vi "get system trace.vi"(6 "Amplifier":T1(ring), 7 "Attenuator":enum16{"NA", "6dB-ME811 "}(ring), 8 "Cable 3":enum16{"NA", "ME1249", "ME1245", "ME1244"}(ring), 9 "Cable 2":enum16{"NA", "ME1249", "ME1245", "ME1244"}(ring), 10 "Cable 1":enum16{"NA", "ME1249", "ME1245", "ME1244"}(ring), 11 "Antenna":T2(ring)) -> (0 "Nuber of Points":i32, 2 "Corrected System Trace":cluster{dbl[], "x+y":dbl[]}, 3 "Corrected 2D array":dbl[][](array[numeric]))   [LabVIEW 2016]
doc: "This VI generate corrected plot of measurement system adding up antenna factor, cable loss, attenuation and amplification along the way."
panel:
  out "Stop Frequency":dbl
  out "Start Frequency":dbl
  out "XY Graph":cluster{dbl[], "x+y":dbl[]}(graph)
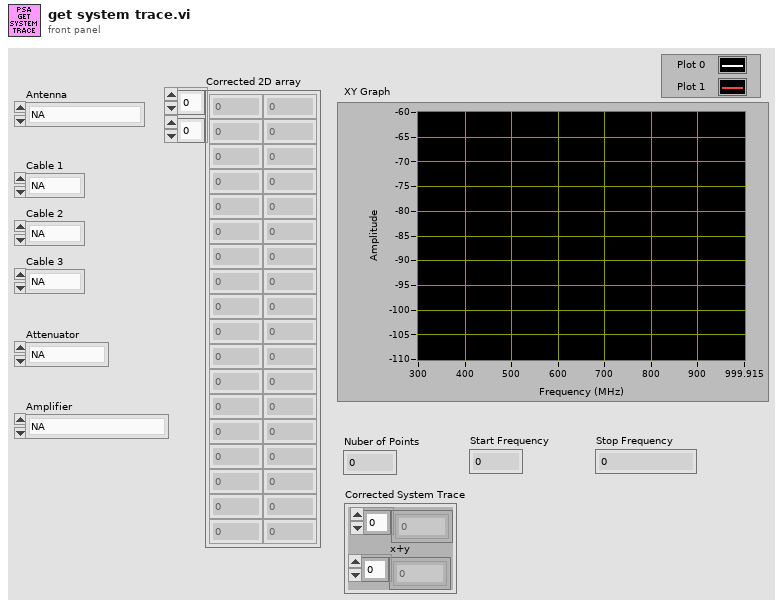
[diagram p1: front panel]
types:
  T1 = enum16{"NA", "500M-18GHz-ME1241", "10K-2GHz-ME813"}
  T2 = enum16{"NA", "ME1284 Periodical", "ME828 Biconical"}
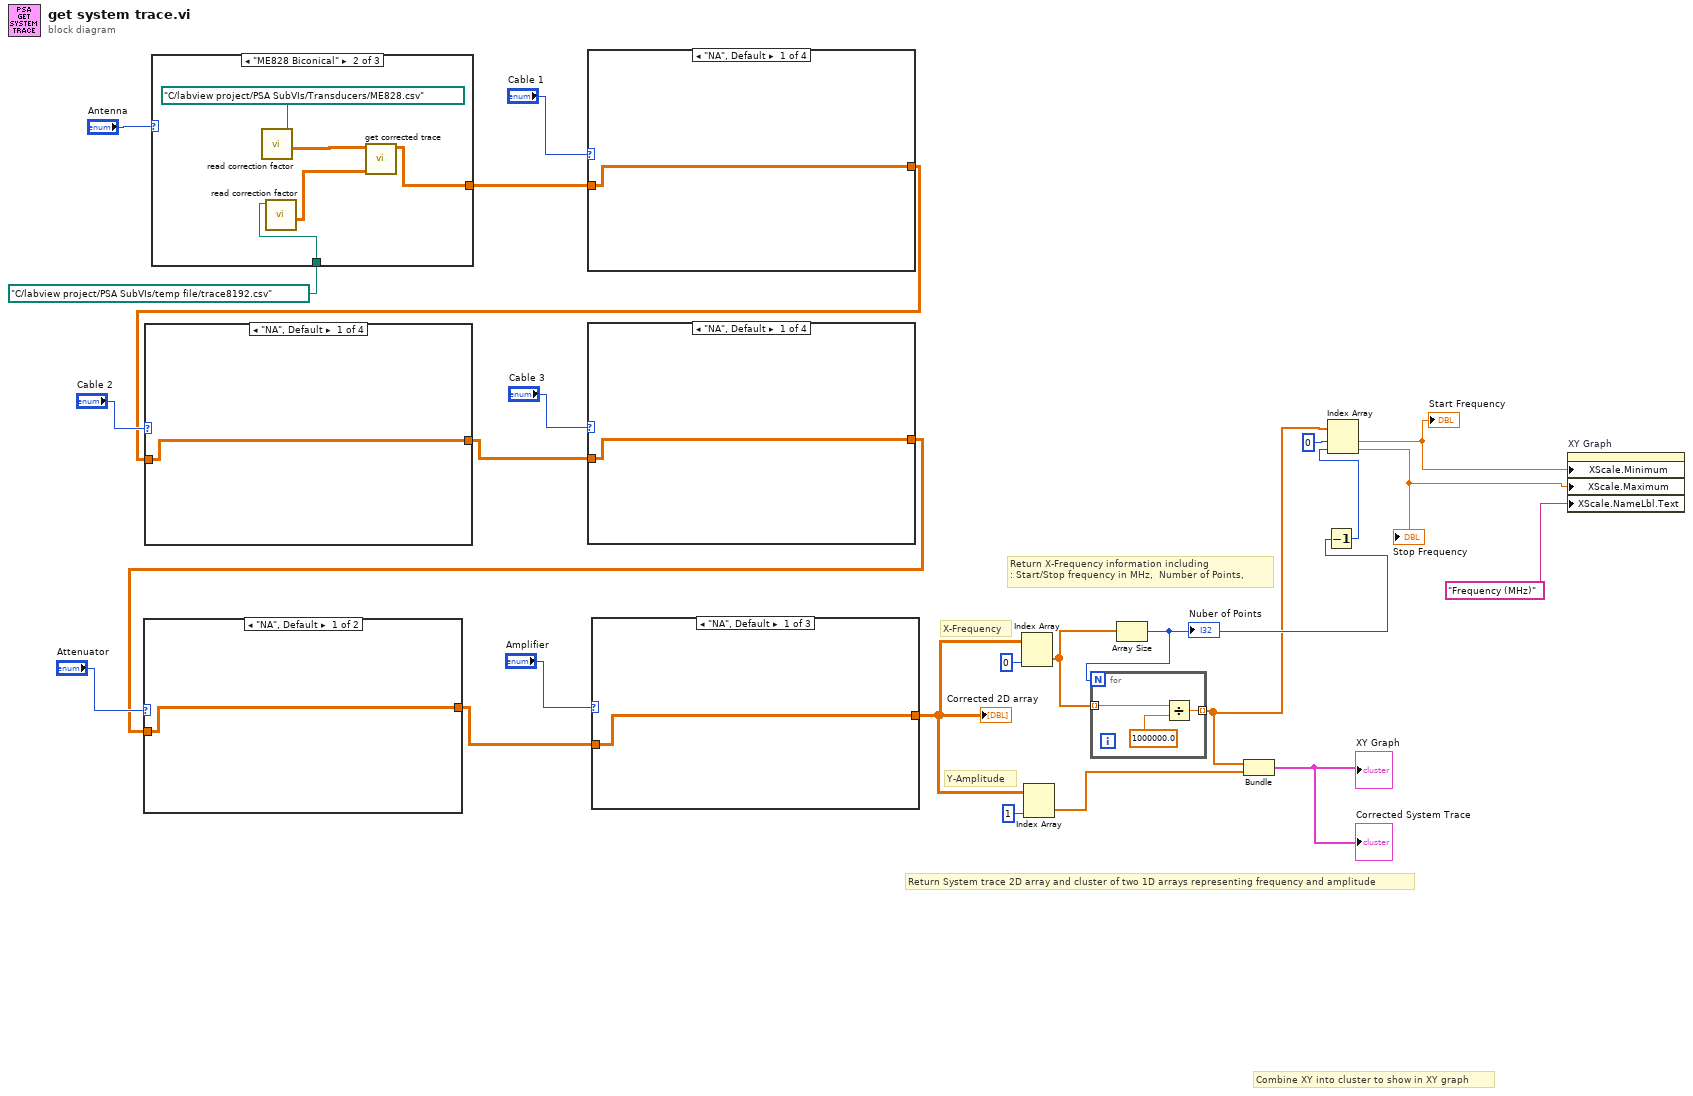
[diagram p0: block diagram]
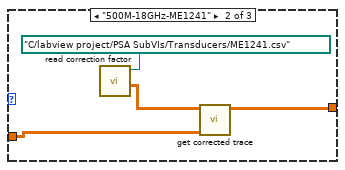
[diagram p2: hidden frame]
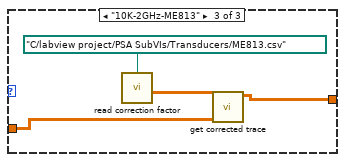
[diagram p3: hidden frame]
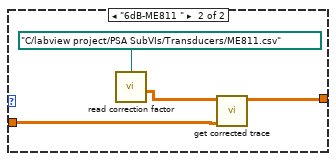
[diagram p4: hidden frame]
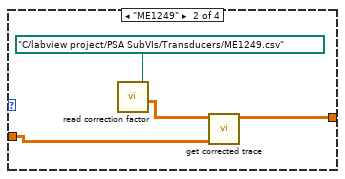
[diagram p5: hidden frame]
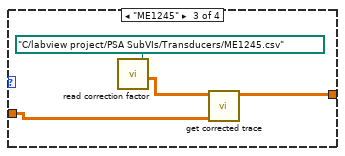
[diagram p6: hidden frame]
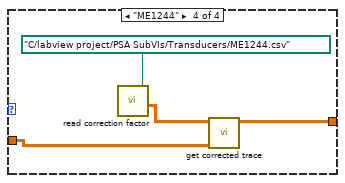
[diagram p7: hidden frame]
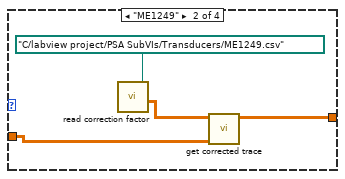
[diagram p8: hidden frame]
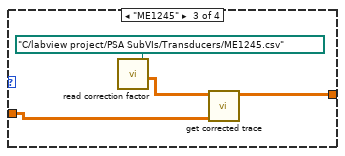
[diagram p9: hidden frame]
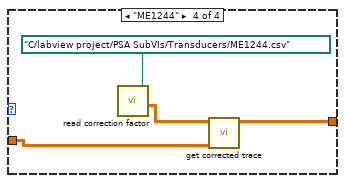
[diagram p10: hidden frame]
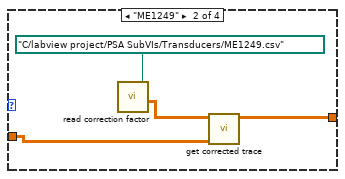
[diagram p11: hidden frame]
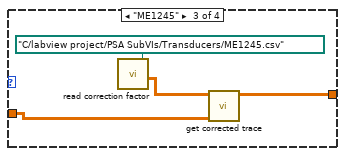
[diagram p12: hidden frame]
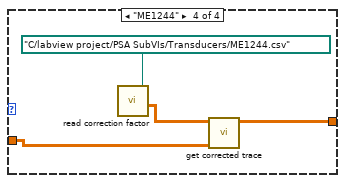
[diagram p13: hidden frame]
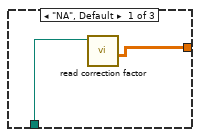
[diagram p14: hidden frame]
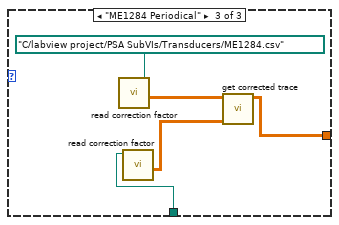
[diagram p15: hidden frame]
diagram:
  # "Return System trace 2D array and cluster of two 1D arrays representing frequency and amplitude"
  # "Combine XY into cluster to show in XY graph"
  # "Return X-Frequency information including\n: Start/Stop frequency in MHz,  Number of Points,"
  # "Y-Amplitude"
  # "X-Frequency"
  n1 = case shown="\"ME828 Biconical\"" "Antenna" {
    tunnel: path "C:/labview project/PSA SubVIs/temp file/trace8192.csv" ("Path") -> [w27 w30 w35]
    tunnel: [w26 w28 w33] -> w22
    frame "NA", Default {
      n2 = call "read correction factor.vi"("Path"=w27) -> ("Output Array"=w26:dbl[][])  [unwired: 7 in, 3 out]
    }
    frame "ME828 Biconical" {
      n3 = call "read correction factor.vi"("Path"=path "C:/labview project/PSA SubVIs/Transducers/ME828.csv") -> ("Output Array"=w32:dbl[][])  [unwired: 7 in, 3 out]
      n4 = call "read correction factor.vi"("Path"=w30) -> ("Output Array"=w29:dbl[][])  [unwired: 7 in, 3 out]
      n5 = call "get corrected trace.vi"("Trace 2D array"=w29, "Transducer 2D array"=w32) -> ("x+y"=w28:dbl[][])  [unwired: 9 in]
    }
    frame "ME1284 Periodical" {
      n6 = call "read correction factor.vi"("Path"=path "C:/labview project/PSA SubVIs/Transducers/ME1284.csv") -> ("Output Array"=w37:dbl[][])  [unwired: 7 in, 3 out]
      n7 = call "read correction factor.vi"("Path"=w35) -> ("Output Array"=w34:dbl[][])  [unwired: 7 in, 3 out]
      n8 = call "get corrected trace.vi"("Trace 2D array"=w34, "Transducer 2D array"=w37) -> ("x+y"=w33:dbl[][])  [unwired: 9 in]
    }
  }
  n9 = case shown="\"NA\", Default" "Cable 1" {
    tunnel: w22 -> [w38 w40 w44 w48]
    tunnel: [w38 w39 w43 w47] -> w20
    frame "NA", Default {
    }
    frame "ME1249" {
      n10 = call "read correction factor.vi"("Path"=path "C:/labview project/PSA SubVIs/Transducers/ME1249.csv") -> ("Output Array"=w41:dbl[][])  [unwired: 7 in, 3 out]
      n11 = call "get corrected trace.vi"("Trace 2D array"=w40, "Transducer 2D array"=w41) -> ("x+y"=w39:dbl[][])  [unwired: 9 in]
    }
    frame "ME1245" {
      n12 = call "read correction factor.vi"("Path"=path "C:/labview project/PSA SubVIs/Transducers/ME1245.csv") -> ("Output Array"=w45:dbl[][])  [unwired: 7 in, 3 out]
      n13 = call "get corrected trace.vi"("Trace 2D array"=w44, "Transducer 2D array"=w45) -> ("x+y"=w43:dbl[][])  [unwired: 9 in]
    }
    frame "ME1244" {
      n14 = call "read correction factor.vi"("Path"=path "C:/labview project/PSA SubVIs/Transducers/ME1244.csv") -> ("Output Array"=w49:dbl[][])  [unwired: 7 in, 3 out]
      n15 = call "get corrected trace.vi"("Trace 2D array"=w48, "Transducer 2D array"=w49) -> ("x+y"=w47:dbl[][])  [unwired: 9 in]
    }
  }
  n16 = case shown="\"NA\", Default" "Cable 2" {
    tunnel: w20 -> [w51 w53 w57 w61]
    tunnel: [w51 w52 w56 w60] -> w18
    frame "NA", Default {
    }
    frame "ME1249" {
      n17 = call "read correction factor.vi"("Path"=path "C:/labview project/PSA SubVIs/Transducers/ME1249.csv") -> ("Output Array"=w54:dbl[][])  [unwired: 7 in, 3 out]
      n18 = call "get corrected trace.vi"("Trace 2D array"=w53, "Transducer 2D array"=w54) -> ("x+y"=w52:dbl[][])  [unwired: 9 in]
    }
    frame "ME1245" {
      n19 = call "read correction factor.vi"("Path"=path "C:/labview project/PSA SubVIs/Transducers/ME1245.csv") -> ("Output Array"=w58:dbl[][])  [unwired: 7 in, 3 out]
      n20 = call "get corrected trace.vi"("Trace 2D array"=w57, "Transducer 2D array"=w58) -> ("x+y"=w56:dbl[][])  [unwired: 9 in]
    }
    frame "ME1244" {
      n21 = call "read correction factor.vi"("Path"=path "C:/labview project/PSA SubVIs/Transducers/ME1244.csv") -> ("Output Array"=w62:dbl[][])  [unwired: 7 in, 3 out]
      n22 = call "get corrected trace.vi"("Trace 2D array"=w61, "Transducer 2D array"=w62) -> ("x+y"=w60:dbl[][])  [unwired: 9 in]
    }
  }
  n23 = case shown="\"NA\", Default" "Cable 3" {
    tunnel: w18 -> [w64 w66 w70 w74]
    tunnel: [w64 w65 w69 w73] -> w16
    frame "NA", Default {
    }
    frame "ME1249" {
      n24 = call "read correction factor.vi"("Path"=path "C:/labview project/PSA SubVIs/Transducers/ME1249.csv") -> ("Output Array"=w67:dbl[][])  [unwired: 7 in, 3 out]
      n25 = call "get corrected trace.vi"("Trace 2D array"=w66, "Transducer 2D array"=w67) -> ("x+y"=w65:dbl[][])  [unwired: 9 in]
    }
    frame "ME1245" {
      n26 = call "read correction factor.vi"("Path"=path "C:/labview project/PSA SubVIs/Transducers/ME1245.csv") -> ("Output Array"=w71:dbl[][])  [unwired: 7 in, 3 out]
      n27 = call "get corrected trace.vi"("Trace 2D array"=w70, "Transducer 2D array"=w71) -> ("x+y"=w69:dbl[][])  [unwired: 9 in]
    }
    frame "ME1244" {
      n28 = call "read correction factor.vi"("Path"=path "C:/labview project/PSA SubVIs/Transducers/ME1244.csv") -> ("Output Array"=w75:dbl[][])  [unwired: 7 in, 3 out]
      n29 = call "get corrected trace.vi"("Trace 2D array"=w74, "Transducer 2D array"=w75) -> ("x+y"=w73:dbl[][])  [unwired: 9 in]
    }
  }
  n30 = case shown="\"NA\", Default" "Attenuator" {
    tunnel: w16 -> [w77 w79]
    tunnel: [w77 w78] -> w14
    frame "NA", Default {
    }
    frame "6dB-ME811 " {
      n31 = call "read correction factor.vi"("Path"=path "C:/labview project/PSA SubVIs/Transducers/ME811.csv") -> ("Output Array"=w80:dbl[][])  [unwired: 7 in, 3 out]
      n32 = call "get corrected trace.vi"("Trace 2D array"=w79, "Transducer 2D array"=w80) -> ("x+y"=w78:dbl[][])  [unwired: 9 in]
    }
  }
  n33 = case shown="\"NA\", Default" "Amplifier" {
    tunnel: w14 -> [w82 w84 w88]
    tunnel: [w82 w83 w87] -> w3
    frame "NA", Default {
    }
    frame "500M-18GHz-ME1241" {
      n34 = call "read correction factor.vi"("Path"=path "C:/labview project/PSA SubVIs/Transducers/ME1241.csv") -> ("Output Array"=w85:dbl[][])  [unwired: 7 in, 3 out]
      n35 = call "get corrected trace.vi"("Trace 2D array"=w84, "Transducer 2D array"=w85) -> ("x+y"=w83:dbl[][])  [unwired: 9 in]
    }
    frame "10K-2GHz-ME813" {
      n36 = call "read correction factor.vi"("Path"=path "C:/labview project/PSA SubVIs/Transducers/ME813.csv") -> ("Output Array"=w89:dbl[][])  [unwired: 7 in, 3 out]
      n37 = call "get corrected trace.vi"("Trace 2D array"=w88, "Transducer 2D array"=w89) -> ("x+y"=w87:dbl[][])  [unwired: 9 in]
    }
  }
  "Corrected 2D array" <- w3
  n38 = Index Array(array=w3, index (col)=0 ("disabled index (col)")) -> (element=w5:dbl[])  [unwired: 1 in]
  n39 = Index Array(array=w3, index (col)=1 ("disabled index (col)")) -> (element=w11:dbl[])  [unwired: 1 in]
  n40 = Array Size(array=w5) -> (size(s)=w4:i32)
  "Nuber of Points" <- w4
  n41 = for {
    N: w4 -> [_]
    tunnel: w5 -> [w92] mode=indexing
    tunnel: [w91] -> w2 mode=indexing
    n42 = Divide(x=w92, y=1000000.0) -> (x/y=w91:dbl)
  }
  n43 = Bundle(w2, "x+y"=w11) -> (→"XY Graph" →"Corrected System Trace":cluster{dbl[], "x+y":dbl[]})  [unwired: 1 in]
  n44 = Decrement(x=w4) -> (x-1=w9:i32)
  n45 = Index Array(array=w2, index #1=0 ("index"), index #2=w9) -> (element #1=w7:dbl, element #2=w6:dbl)
  "Start Frequency" <- w7
  "Stop Frequency" <- w6
  n46 = property on="XY Graph" class="XYGraph (strict)"("XScale.Minimum"=w7, "XScale.Maximum"=w6, "XScale.NameLbl.Text"="Frequency (MHz)" ("X Scale.Unit Label.Text")) -> ()  [unwired: 2 in, 2 out]
